vi "analizador de vibraciones.vi"() -> ()   [LabVIEW 2014]
panel:
  out "Z":dbl[](graph)
  out "Y":dbl[](graph)
  out "X":dbl[](graph)
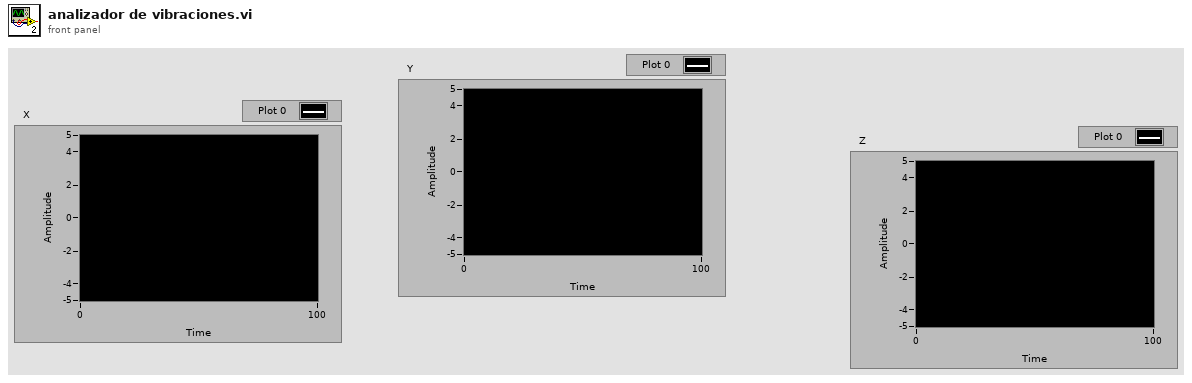
[diagram p1: front panel]
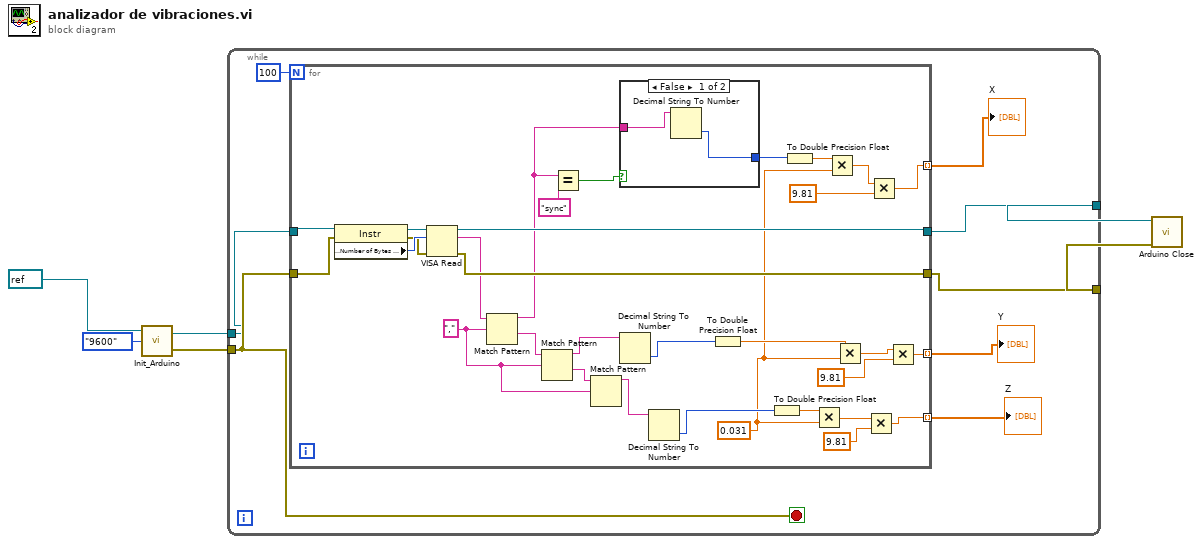
[diagram p0: block diagram]
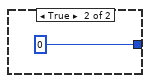
[diagram p2: hidden frame]
diagram:
  n1 = call "Init_Arduino.vi"("Velocidad de Conexion"=enum16{"115200", "9600"}."9600", "VISA Refnum in"=refnum<visa-resource-name> refnum) -> ("error out"=w6:errorcluster, "VISA Refnum out"=w5:refnum<visa-resource-name>)  [unwired: 1 in]
  n2 = while {
    tunnel: w6 -> [w14]
    tunnel: w5 -> [w13]
    tunnel: [w12] -> w2
    tunnel: [w11] -> w1
    stop <- w14 stop-if-true
    n3 = for {
      N: 100 -> [_]
      tunnel: w14 -> [w15]
      tunnel: [w45] -> w11
      tunnel: w13 -> [w16]
      tunnel: [w46] -> w12
      tunnel: [w20] -> w8 mode=indexing
      tunnel: [w21] -> w7 mode=indexing
      tunnel: [w28] -> w9 mode=indexing
      w29 = 0.031 ("y")
      w43 = "," ("regular expression")
      n4 = property class="Instr"(reference=w16, error in=w15) -> (reference out=w17:refnum<visa-resource-name>, error out=w18:errorcluster, "Serial Settings:Number of Bytes at Serial Port"=w19:u32)
      n5 = VISA Read(VISA resource name=w17, byte count=w19, error in (no error)=w18) -> (VISA resource name out=w46:refnum<visa-resource-name>, read buffer=w44:string, error out=w45:errorcluster)  [unwired: 1 out]
      n6 = Match Pattern(string=w44, regular expression=w43) -> (before substring=w38:string, after substring=w42:string)  [unwired: 1 in, 2 out]
      n7 = Match Pattern(string=w42, regular expression=w43) -> (before substring=w37:string, after substring=w41:string)  [unwired: 1 in, 2 out]
      n8 = Equal?(x=w38, y="sync") -> (x = y?=w39:bool)
      n9 = Match Pattern(string=w41, regular expression=w43) -> (before substring=w36:string)  [unwired: 1 in, 3 out]
      n10 = case shown="False" w39 {
        tunnel: [w47 0] -> w35
        tunnel: w38 -> [w48 _]
        frame False {
          n11 = Decimal String To Number(string=w48) -> (number=w47:i32)  [unwired: 2 in, 1 out]
        }
        frame True {
        }
      }
      n12 = Decimal String To Number(string=w37) -> (number=w32:i32)  [unwired: 2 in, 1 out]
      n13 = Decimal String To Number(string=w36) -> (number=w30:i32)  [unwired: 2 in, 1 out]
      n14 = To Double Precision Float(number=w32) -> (double precision float=w33:dbl)
      n15 = To Double Precision Float(number=w30) -> (double precision float=w31:dbl)
      n16 = To Double Precision Float(number=w35) -> (double precision float=w34:dbl)
      n17 = Multiply(x=w31, y=w29) -> (x*y=w27:dbl)
      n18 = Multiply(x=w34, y=w29) -> (x*y=w25:dbl)
      n19 = Multiply(x=w33, y=w29) -> (x*y=w26:dbl)
      n20 = Multiply(x=w27, y=9.81) -> (x*y=w28:dbl)
      n21 = Multiply(x=w25, y=9.81) -> (x*y=w20:dbl)
      n22 = Multiply(x=w26, y=9.81) -> (x*y=w21:dbl)
    }
    "Z" <- w9
    "X" <- w8
    "Y" <- w7
  }
  n23 = call "Arduino Close.vi"("error in (no error)"=w1, "VISA Refnum in"=w2) -> ()  [unwired: 10 in]
